vi "getObject.vi"(1 "bentStyle":T1, 5 "error in (no error)":errorcluster) -> (14 "reference out":refnum<class "BentStyle.lvclass">, 19 "error out":errorcluster)   [LabVIEW 2016, in "BentStyle.lvclass"]
doc: "Gets a specific object"
uses:
  <resource>/Framework/Providers/Open_GDS/UML/BentStyle_class/BentStyle.lvclass
  <resource>/Framework/Providers/Open_GDS/UML/BentStyle_class/BentStyleType.ctl
  <resource>/Framework/Providers/Open_GDS/UML/BentStyle_class/BentStyle.lvclass/BentStyle.ctl
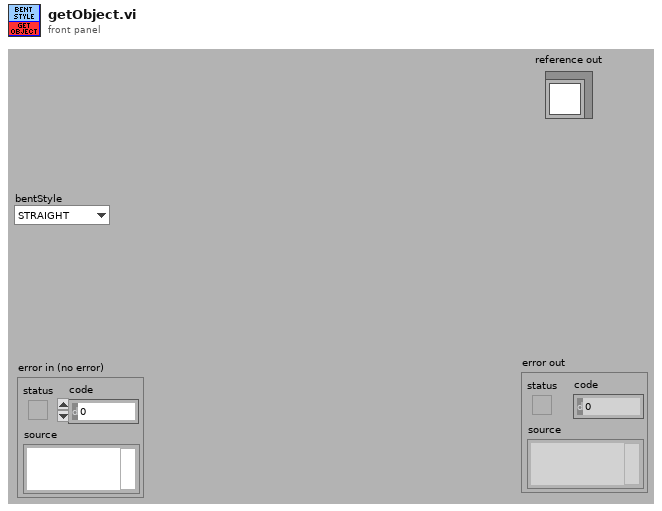
[diagram p1: front panel]
types:
  T1 = typedef "BentStyle.lvclass/BentStyleType.ctl" = enum16{"STRAIGHT", "HV", "VH", "HVH", "VHV", "ARC"}
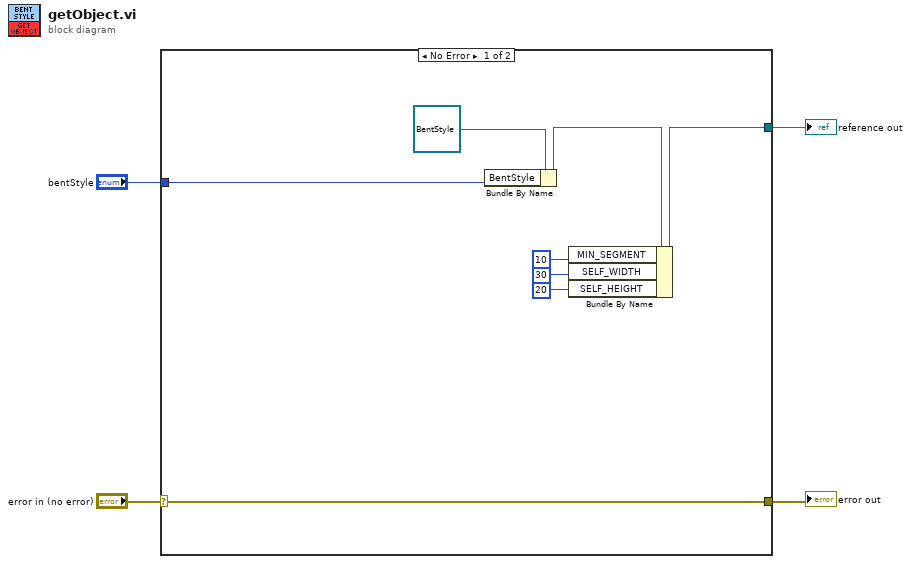
[diagram p0: block diagram]
diagram:
  n1 = case shown="No Error" "error in (no error)" {
    selector: "error in (no error)" -> [w10 w13]
    tunnel: [w10 w13] -> w3
    tunnel: [w5 _] -> w2
    tunnel: "bentStyle" -> [w11 _]
    frame No Error {
      n2 = Bundle By Name(cluster=refnum<class "BentStyle.lvclass"> refnum ("ARC"), "BentStyle"=w11) -> (w6:refnum<class "BentStyle.lvclass">)
      n3 = Bundle By Name(cluster=w6, "MIN_SEGMENT"=10, "SELF_WIDTH"=30, "SELF_HEIGHT"=20) -> (w5:refnum<class "BentStyle.lvclass">)
    }
    frame Error {
    }
  }
  "error out" <- w3
  "reference out" <- w2
